vi "Broadcast Response.vi"(8 "error in (no error)":errorcluster, 9 "Acquired Result.lvclass":refnum<class "Acquired Result.lvclass">, 10 "Topic":string, 11 "Integrate in":refnum<class "Integrate.lvclass">) -> (0 "error out":errorcluster, 3 "Integrate out":refnum<class "Integrate.lvclass">)   [LabVIEW 2015, in "Integrate.lvclass"]
uses:
  Integrate.lvclass
  Measure_core/Results/Acquired Result/Acquired Result.lvclass
  <vilib>/ActorFramework/Actor/Actor.lvclass/Actor.ctl
  Monitor-Pulse Messages/Write Peak Field Msg/Write Peak Field Msg.lvclass/Write Peak Field Msg.ctl
  <vilib>/ActorFramework/Message Enqueuer/Message Enqueuer.lvclass/Message Enqueuer.ctl
  <vilib>/ActorFramework/Message Enqueuer/Enqueue.vi
  Read Integrate Configuration.vi
  <vilib>/ActorFramework/Message Priority Queue/Priority Enqueue.vi
  Monitor-Pulse Messages/Write Peak Field Msg/Write Peak Field Msg.lvclass
  <vilib>/ActorFramework/Actor/Actor.lvclass
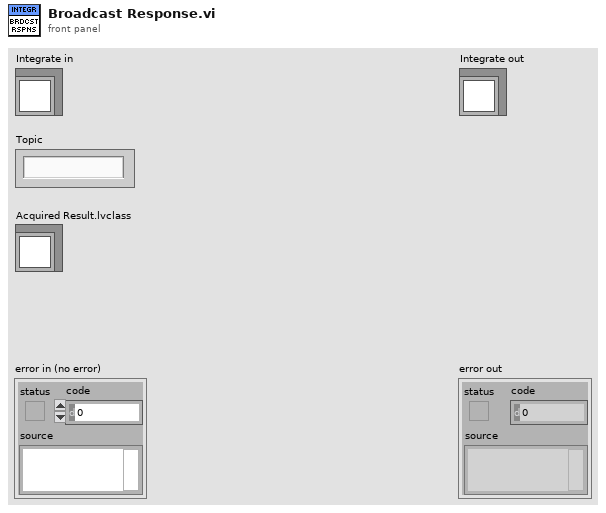
[diagram p1: front panel]
types:
  T1 = typedef "Integrator Configoration.ctl" = cluster{"Integrate":T2[], "Offset duration ":dbl, "TDMS group name":string}
  T2 = typedef "Integrate channel.ctl" = cluster{"Channel":string, "Output name":string, "Factor":dbl, "Start time":dbl, "Duration":dbl}
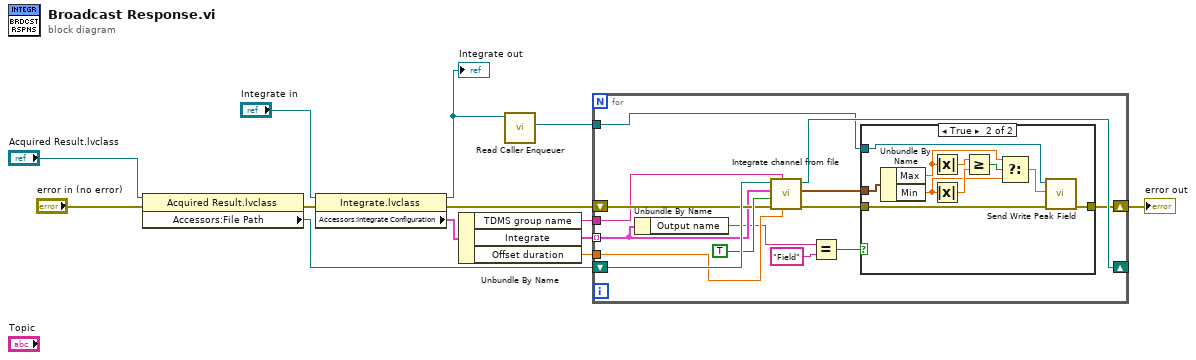
[diagram p0: block diagram]
diagram:
  n1 = property class="Acquired Result.lvclass"(reference="Acquired Result.lvclass", error in="error in (no error)") -> (error out=w7:errorcluster, "Accessors:File Path"=w9:path)  [unwired: 1 out]
  n2 = property class="Integrate.lvclass"(reference="Integrate in", error in=w7) -> (reference out=w3:refnum<class "Integrate.lvclass">, error out=w8:errorcluster, "Accessors:Integrate Configuration"=w11:T1)
  "Integrate out" <- w3
  n3 = Unbundle By Name(w11) -> ("TDMS group name"=w1:string, "Integrate"=w10:T2[], "Offset duration"=w5:dbl)
  n4 = call <vilib>:"Read Caller Enqueuer.vi"("Actor"=w3) -> ("Caller Enqueuer"=w2:refnum<class "Message Enqueuer.lvclass">)  [unwired: 10 in]
  n5 = for {
    tunnel: w10 -> [w22] mode=indexing
    shift-right: [w26] -> _
    shift-left: w9 -> [w27]
    tunnel: w5 -> [w23]
    shift-right: [w17] -> w4
    shift-left: w8 -> [w24]
    tunnel: w2 -> [w16]
    tunnel: w1 -> [w14]
    n6 = Unbundle By Name(w22) -> ("Output name"=w21:string)
    n7 = call "Integrate channel from file.vi"("Offset duration"=w23, "group name in"=w14, "Error In"=w24, "Save data"=TRUE, "Integration settings"=w22, "File Path Control"=w27) -> ("Error Out"=w18:errorcluster, "Min max"=w15:cluster{"Max":dbl, "Min":dbl}, "File Path out"=w26:path)  [unwired: 2 in, 1 out]
    n8 = Equal?(x=w21, y="Field") -> (x = y?=w19:bool)
    n9 = case shown="True" w19 {
      tunnel: w18 -> [w28 w38]
      tunnel: [w28 w37] -> w17
      tunnel: w16 -> [_ w36]
      tunnel: w15 -> [_ w35]
      frame False {
      }
      frame True {
        n10 = Unbundle By Name(w35) -> ("Max"=w32:dbl, "Min"=w29:dbl)
        n11 = Absolute Value(x=w32) -> (abs(x)=w31:dbl)
        n12 = Absolute Value(x=w29) -> (abs(x)=w30:dbl)
        n13 = Greater Or Equal?(x=w31, y=w30) -> (x >= y?=w34:bool)
        n14 = Select(t=w32, s=w34, f=w29) -> (s? t:f=w33:dbl)
        n15 = call "Send Write Peak Field.vi"("error in (no error)"=w38, "Peak Field"=w33, "Message Enqueuer"=w36) -> ("error out"=w37:errorcluster)  [unwired: 7 in, 1 out]
      }
    }
  }
  "error out" <- w4
